vi "Ballard XML Generator.Add Parameter Properties Multiple.vi"(0 "string in":string, 1 "Channel Number":i32, 7 "Parameter Array":T1[](array[typedef])) -> (4 "string out":string)   [LabVIEW 2017]
uses:
  Controls/Database_Array.ctl
  Controls/Encoding.ctl
  <userlib>/_OpenG.lib/array/array.llb/Search 1D Array (I16)__ogtk.vi
  <userlib>/_OpenG.lib/array/array.llb/Index 1D Array Elements (Variant)__ogtk.vi
  <userlib>/_OpenG.lib/array/array.llb/Sort 1D Array (I32)__ogtk.vi
  <userlib>/_OpenG.lib/array/array.llb/Index 1D Array Elements (String)__ogtk.vi
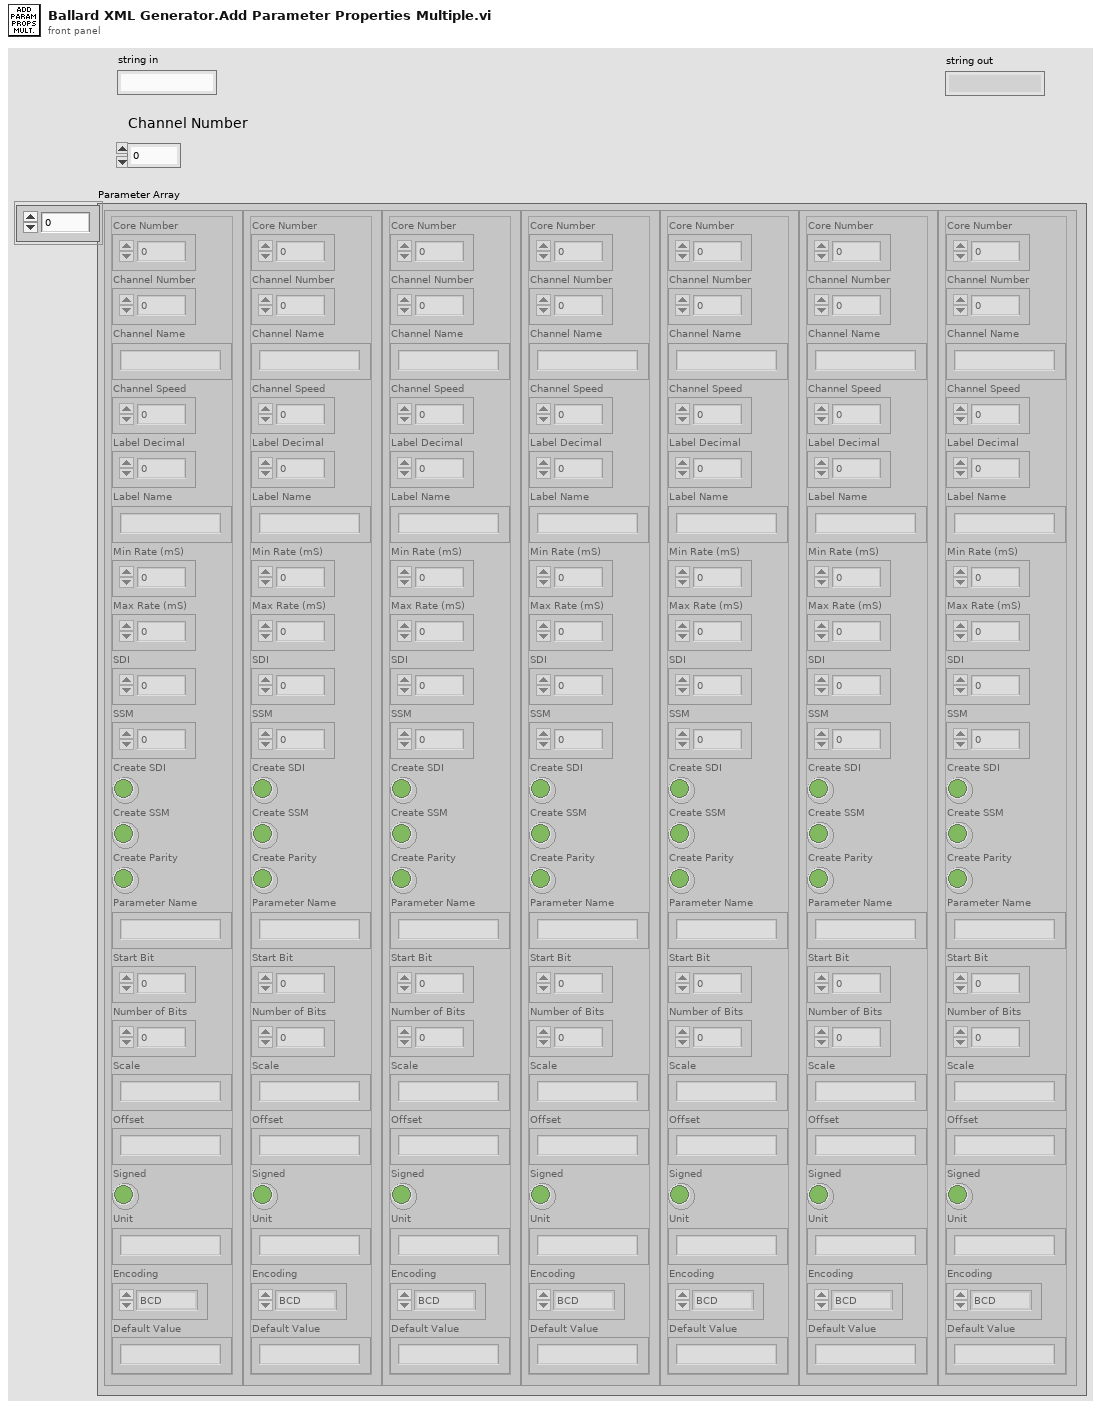
[diagram p1: front panel]
types:
  T1 = typedef "Database_Array.ctl" = cluster{"Core Number":i32, "Channel Number":i32, "Channel Name":string, "Channel Speed":i32, "Label Decimal":i32, "Label Name":string, "Min Rate (mS)":i32, "Max Rate (mS)":i32, "SDI":i32, "SSM":i32, "Create SDI":bool, "Create SSM":bool, "Create Parity":bool, "Parameter Name":string, "Start Bit":i32, "Number of Bits":i32, "Scale":string, "Offset":string, "Signed":bool, "Unit":string, "Encoding":T2, "Default Value":string}
  T2 = typedef "Encoding.ctl" = enum16{"BCD", "BNR", "Discrete"}
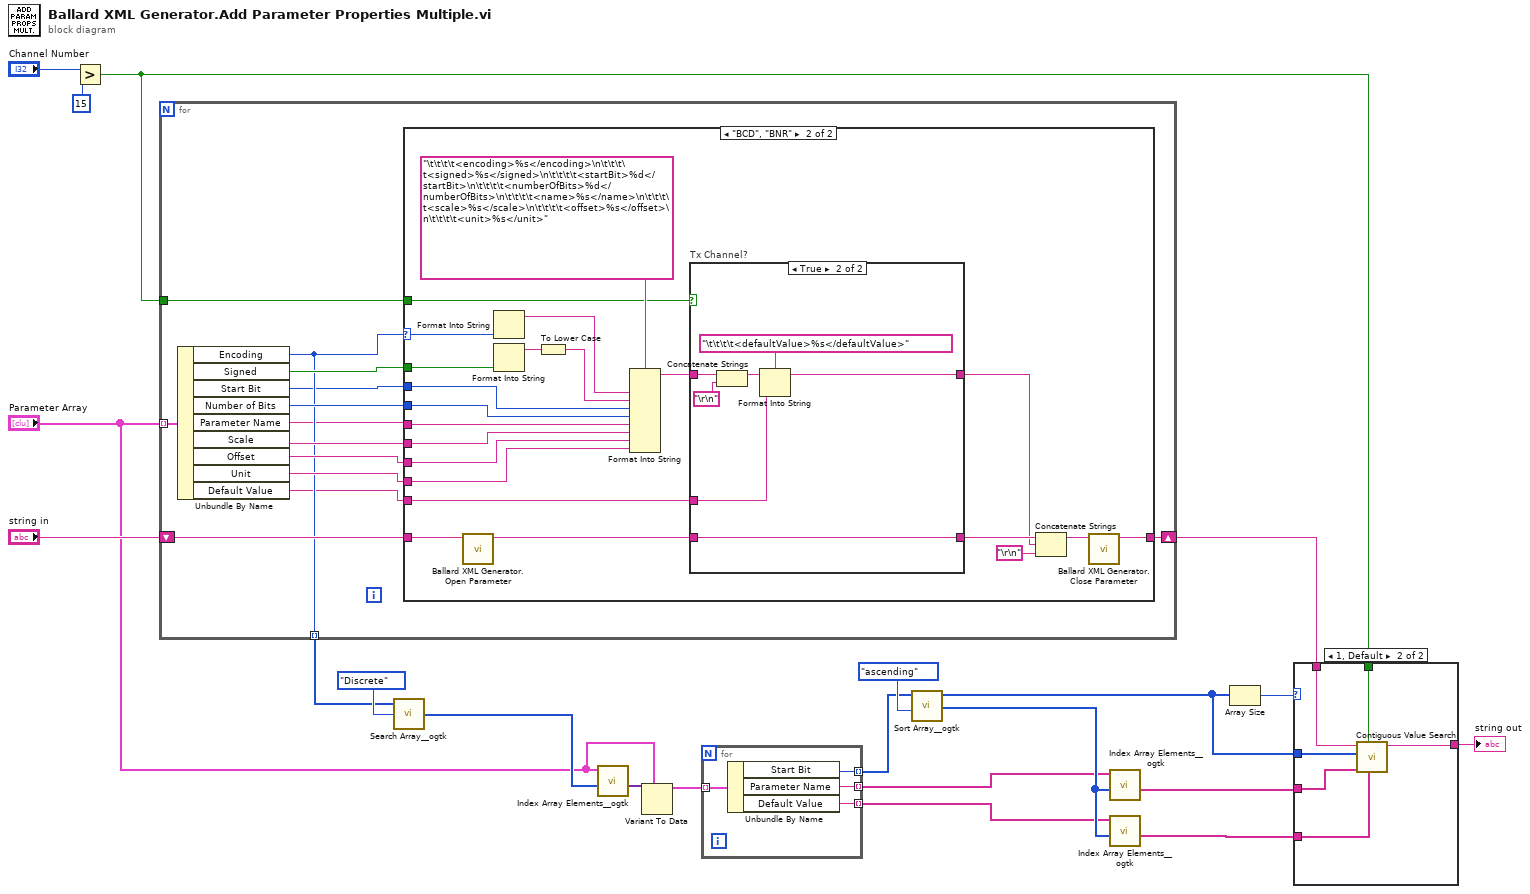
[diagram p0: block diagram]
diagram:
  n1 = Greater?(x="Channel Number", y=15) -> (0:w10:bool)
  n2 = for {
    shift-right: [w33] -> w17
    shift-left: "string in" -> [w34]
    tunnel: w10 -> [w32]
    tunnel: "Parameter Array" -> [w31] mode=indexing
    tunnel: [w25] -> w8 mode=indexing
    n3 = Unbundle By Name(w31) -> ("Encoding"=w25:T2, "Signed"=w30:bool, "Start Bit"=w24:i32, "Number of Bits"=w29:i32, "Parameter Name"=w23:string, "Scale"=w28:string, "Offset"=w27:string, "Unit"=w26:string, "Default Value"=w22:string)
    n4 = case shown="\"BCD\", \"BNR\"" w25 {
      selector: w25 -> [_ w47]
      tunnel: w30 -> [_ w57]
      tunnel: w26 -> [_ w55]
      tunnel: w27 -> [_ w54]
      tunnel: w28 -> [_ w53]
      tunnel: w23 -> [_ w52]
      tunnel: w29 -> [_ w51]
      tunnel: w24 -> [_ w50]
      tunnel: w22 -> [_ w42]
      tunnel: w34 -> [w35 w46]
      tunnel: [w35 w44] -> w33
      tunnel: w32 -> [_ w40]
      frame "Discrete", Default {
      }
      frame "BCD", "BNR" {
        n5 = call "Ballard XML Generator.Open Parameter.vi"("string in"=w46) -> ("string out"=w45:string)  [unwired: 10 in]
        n6 = Format Into String(w47) -> (resulting string=w48:string)  [unwired: 3 in, 1 out]
        n7 = Format Into String(w57) -> (resulting string=w56:string)  [unwired: 3 in, 1 out]
        n8 = To Lower Case(string=w56) -> (all lower case string=w49:string)
        n9 = Format Into String(format string="\t\t\t\t<encoding>%s</encoding>\n\t\t\t\t<signed>%s</signed>\n\t\t\t\t<startBit>%d</startBit>\n\t\t\t\t<numberOfBits>%d</numberOfBits>\n\t\t\t\t<name>%s</name>\n\t\t\t\t<scale>%s</scale>\n\t\t\t\t<offset>%s</offset>\n\t\t\t\t<unit>%s</unit>", w48, w49, w50, w51, w52, w53, w54, w55) -> (resulting string=w41:string)  [unwired: 2 in, 1 out]
        n10 = case "Tx Channel?" shown="True" w40 {
          tunnel: w45 -> [w59 w64]
          tunnel: w42 -> [_ w65]
          tunnel: w41 -> [w58 w62]
          tunnel: [w59 w64] -> w38
          tunnel: [w58 w63] -> w37
          frame False {
          }
          frame True {
            n11 = Concatenate Strings(w62, "\r\n") -> (w61:string)
            n12 = Format Into String(format string="\t\t\t\t<defaultValue>%s</defaultValue>", initial string=w61, w65) -> (resulting string=w63:string)  [unwired: 1 in, 1 out]
          }
        }
        n13 = Concatenate Strings(w38, w37, "\r\n") -> (w36:string)
        n14 = call "Ballard XML Generator.Close Parameter.vi"("string in"=w36) -> ("string out"=w44:string)  [unwired: 10 in]
      }
    }
  }
  n15 = call-poly <userlib>:"Search Array__ogtk.vi"("Array"=w8, "Element Data"=Encoding."Discrete" ("encoding (BNR)")) -> ("Indices of Elements"=w7:i32[])  [unwired: 7 in]
  n16 = call-poly <userlib>:"Index Array Elements__ogtk.vi"("indices"=w7, "array"="Parameter Array") -> ("elements"=w6:variant[])  [unwired: 9 in]
  n17 = Variant To Data(type="Parameter Array", Variant=w6) -> (data=w4:T1[])  [unwired: 1 in, 1 out]
  n18 = for {
    tunnel: w4 -> [w70] mode=indexing
    tunnel: [w69] -> w3 mode=indexing
    tunnel: [w68] -> w2 mode=indexing
    tunnel: [w67] -> w1 mode=indexing
    n19 = Unbundle By Name(w70) -> ("Start Bit"=w67:i32, "Parameter Name"=w69:string, "Default Value"=w68:string)
  }
  n20 = call-poly <userlib>:"Sort Array__ogtk.vi"("Order"=enum16{"ascending", "descending"}."ascending", "Array in"=w1) -> ("Sorted Pointers"=w19:i32[], "Sorted Array out"=w16:i32[])  [unwired: 8 in]
  n21 = call-poly <userlib>:"Index Array Elements__ogtk.vi"("indices"=w19, "array"=w3) -> ("elements"=w18:string[])  [unwired: 9 in]
  n22 = call-poly <userlib>:"Index Array Elements__ogtk.vi"("indices"=w19, "array"=w2) -> ("elements"=w13:string[])  [unwired: 9 in]
  n23 = Array Size(array=w16) -> (size(s)=w15:i32)
  n24 = case shown="1, Default" w15 {
    tunnel: w18 -> [_ w72]
    tunnel: w17 -> [w71 w77]
    tunnel: w16 -> [_ w75]
    tunnel: w10 -> [_ w74]
    tunnel: [w71 w76] -> w14
    tunnel: w13 -> [_ w73]
    frame 0 {
    }
    frame 1, Default {
      n25 = call "Contiguous Value Search.vi"("Sorted Default Value (in)"=w73, "Tx?"=w74, "Sorted Name (in)"=w72, "Sorted Array (in)"=w75, "String (in)"=w77) -> ("String (out)"=w76:string)  [unwired: 6 in]
    }
  }
  "string out" <- w14
